vi "Periodic Tasks.vi"(8 "error in (no error)":errorcluster) -> ()   [LabVIEW 2014]
doc: "This VI runs in parallel to other tasks. It can contain as many user-defined periodic loops as you need. These can carry out PID or other sorts of timed response."
uses:
  Variables/References.vi
  <vilib>/Rock Robotics/SystemInterfaces/Utilities/FPGA_UtilitiesRead LocalTime.vi
  Variables/Physical data.vi
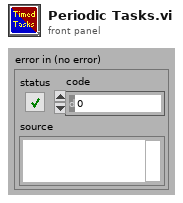
[diagram p1: front panel]
types:
  T1 = typedef "WPI_MotorControlDeviceRef.ctl" = cluster{"DeviceStatus":errorcluster, "Type":T2, "PWM":cluster{"Controller":T3, "PWM Channel":T4, "DeadBand":T5}, "CAN":cluster{"Device Number":u8, "Control Mode":T6, "Semaphore":T7, "Max Vout":dbl, "TalonSRX Control Mode":T8}, "Invert":bool, "TransformRef":T9, "InvTransformRef":T9}
  T2 = typedef "WPI_MotorControlType.ctl" = enum16{"PWM", "CAN", "CANTalonSRX"}
  T3 = typedef "FPGA_TypedefDigitalModule.ctl" = enum16{"Controller 1"}
  T4 = typedef "FPGA_DIOPWMChannel.ctl" = enum8{"PWM 0", "PWM 1", "PWM 2", "PWM 3", "PWM 4", "PWM 5", "PWM 6", "PWM 7", "PWM 8", "PWM 9", "PWM MXP 0", "PWM MXP 1", "PWM MXP 2", "PWM MXP 3", "PWM MXP 4", "PWM MXP 5", "PWM MXP 6", "PWM MXP 7", "PWM MXP 8", "PWM MXP 9", "Invalid"}
  T5 = typedef "WPI_PWMDeadband.ctl" = cluster{"Name":string, "maxPositivePwm":i32, "minPositivePwm":i32, "centerPwm":i32, "maxNegativePwm":i32, "minNegativePwm":i32, "angularRange":u16}
  T6 = typedef "WPI_CANJaguar_ControlMode.ctl" = enum8{"Percent VBus", "Current", "Speed", "Position", "Voltage"}
  T7 = typedef "Semaphore RefNum" = refnum<k1>
  T8 = typedef "WPI_CANTalonSRX_APIControlMode.ctl" = enum8{"Percent VBus", "Speed", "Position", "Slave", "Unchanged / Invalid"}
  T9 = typedef "WPI_PWMTransform_ConPane.ctl" = refnum<vi>
  T10 = typedef "WPI_AnalogChannelDevRef.ctl" = cluster{"DevStatus":errorcluster, "Controller":T11, "Analog Channel":T12}
  T11 = typedef "FPGA_TypedefAnalogModule.ctl" = enum16{"Controller 1"}
  T12 = typedef "FPGA_AIChannel.ctl" = enum8{"AI 0", "AI 1", "AI 2", "AI 3", "AI MXP 0", "AI MXP 1", "AI MXP 2", "AI MXP 3", "Invalid"}
  T13 = typedef "WPI_EncoderDevRef.ctl" = cluster{"DevStatus":errorcluster, "EncoderIndex":T14, "CounterIndex":T15, "DistancePerCount":dbl, "Decoding Type":T16}
  T14 = typedef "FPGA_EncoderIdx.ctl" = enum8{"Enc 0", "Enc 1", "Enc 2", "Enc 3", "Enc 4", "Enc 5", "Enc 6", "Enc 7", "Invalid"}
  T15 = typedef "FPGA_CounterCtrSystemIndex.ctl" = enum8{"Ctr 0", "Ctr 1", "Ctr 2", "Ctr 3", "Ctr 4", "Ctr 5", "Ctr 6", "Ctr 7", "Invalid"}
  T16 = typedef "WPI_EncoderType.ctl" = enum16{"1x", "2x", "4x"}
  T17 = cluster{"DriveMotorRef":T1, "TurretMotorRef":T1, "Turret Encoder":cluster{"AIDeviceRef":T10, "Turret Analog Location":enum16{"RoboRio", "Drive SRX", "Turret SRX"}}, "Drive Encoder":cluster{"EncoderDevRef":T13, "Drive Encoder Location":enum16{"RoboRio", "Drive SRX", "Turret SRX"}}, "Pod position (RCS)":cluster{"X":dbl, "Y":dbl, "Z":dbl}, "Data":cluster{"Drive Motor Output":dbl, "Turret Motor Output":dbl, "Wheel RPM":dbl, "Turret Angle":dbl, "Turret angle offset":dbl, "Transmission moment of inertia":dbl, "Transmission efficiency":dbl, "Wheel dist / rev":dbl, "Turret moment of inertia":dbl, "Inv. turret encoder":bool, "Inv. drive encoder":bool}}[]
  T18 = typedef "NI_Matrix.lvlib/RealMatrix.ctl" = dbl[][]
  T19 = cluster{"All pods":cluster{"Drive":cluster{"Drive Motor Output":dbl, "Wheel RPM":dbl, "Linear speed":dbl, "Linear acceleration":dbl, "Encoder Output":dbl}, "Turret":cluster{"Turret Motor Output":dbl, "Turret Angle":dbl, "Turret velocity":dbl, "Turret acceleration":dbl, "Encoder Output":dbl}, "Pod position (RCS)":cluster{"X":dbl, "Y":dbl, "Z":dbl}}[], "Global Robot Data":cluster{"Position Data":cluster{"Robot Position":cluster{"X":dbl, "Y":dbl, "Z":dbl}, "Robot Velocity":cluster{"X":dbl, "Y":dbl, "Z":dbl}, "Robot Acceleration":cluster{"X":dbl, "Y":dbl, "Z":dbl}}, "Rotation Data":cluster{"Angular Position":cluster{"X":dbl, "Y":dbl, "Z":dbl}, "Angular Velocity":cluster{"X":dbl, "Y":dbl, "Z":dbl}, "Angular Acceleration":cluster{"X":dbl, "Y":dbl, "Z":dbl}}}, "Inertial Characteristics":cluster{"Center of Mass (RCS)":cluster{"X":dbl, "Y":dbl, "Z":dbl}, "Mass Elements":cluster{"X":dbl, "Y":dbl, "Z":dbl, "Mass":dbl, "Name":string}[], "Center of Rotation (RCS)":cluster{"X":dbl, "Y":dbl, "Z":dbl}, "Tensor of Inertia":T18}}
  T20 = cluster{"Drive":cluster{"Drive Motor Output":dbl, "Wheel RPM":dbl, "Linear speed":dbl, "Linear acceleration":dbl, "Encoder Output":dbl}, "Turret":cluster{"Turret Motor Output":dbl, "Turret Angle":dbl, "Turret velocity":dbl, "Turret acceleration":dbl, "Encoder Output":dbl}, "Pod position (RCS)":cluster{"X":dbl, "Y":dbl, "Z":dbl}}
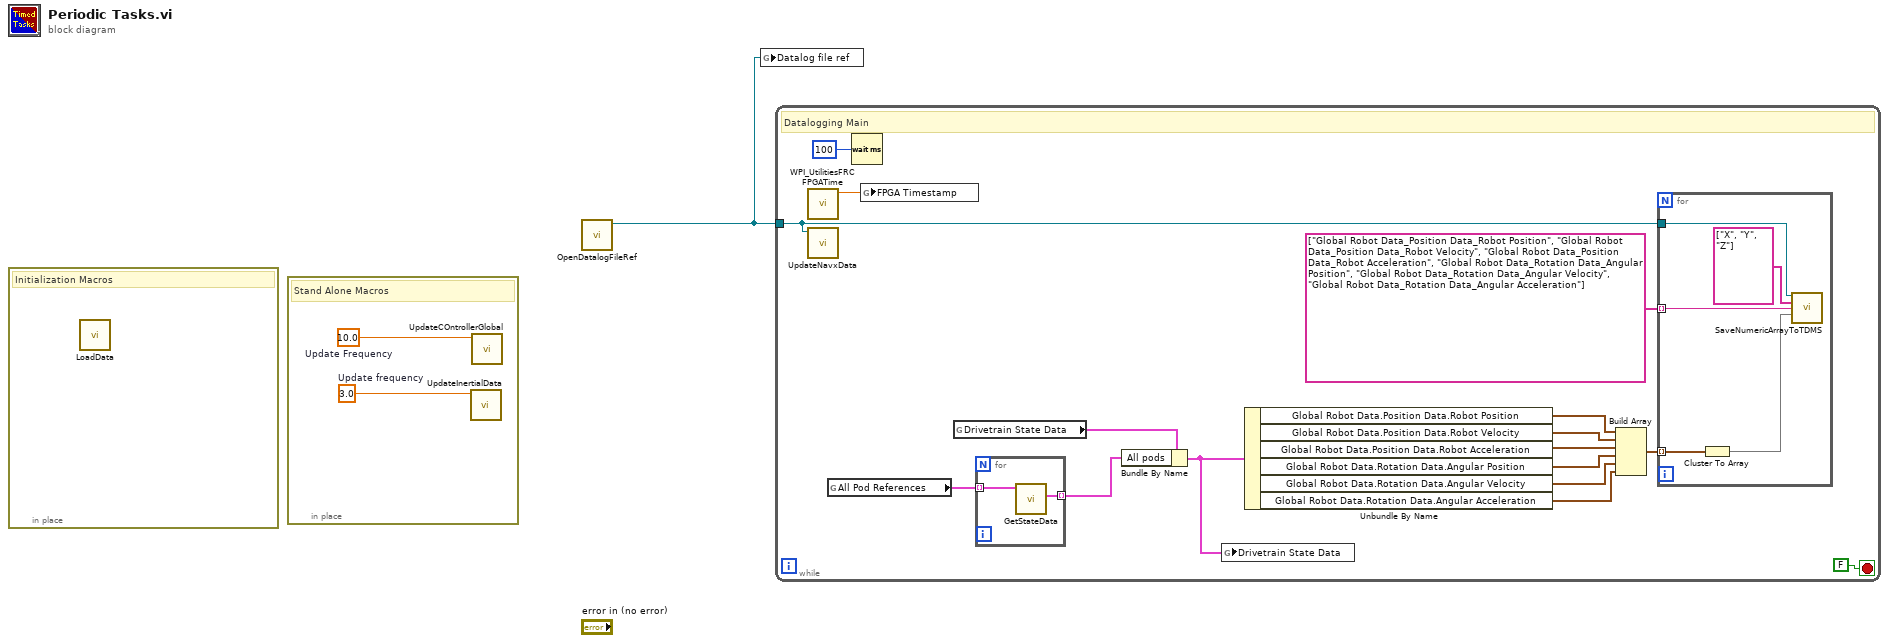
[diagram p0: block diagram]
diagram:
  n1 = in-place {
    # "Initialization Macros"
    n2 = call "LoadData.vi"() -> ()  [unwired: 12 in]
  }
  n3 = in-place {
    w2 = 3.0  # Update frequency
    w3 = 10.0  # Update Frequency
    # "Stand Alone Macros"
    n4 = call "UpdateInertialData.vi"("Update frequency"=w2) -> ()  [unwired: 11 in]
    n5 = call "UpdateCOntrollerGlobal.vi"("Update Frequency"=w3) -> ()  [unwired: 11 in]
  }
  n6 = call "OpenDatalogFileRef.vi"() -> ("tdms file out"=w1:refnum<k34>)  [unwired: 9 in, 2 out]
  n7 = global write "References.vi" "Datalog file ref"(w1) -> ()
  n8 = while {
    tunnel: w1 -> [w4]
    stop <- FALSE stop-if-true
    # "Datalogging Main"
    n9 = call <vilib>:"WPI_UtilitiesFRC FPGATime.vi"() -> ("FPGA Time"=w13:dbl)  [unwired: 10 in, 1 out]
    n10 = call "UpdateNavxData.vi"("Datalogging File Refnum in"=w4) -> ()  [unwired: 11 in]
    n11 = global read "References.vi" "All Pod References"() -> (w18:T17)
    n12 = Wait (ms)(milliseconds to wait=u32 100) -> ()  [unwired: 1 out]
    n13 = global write "Physical data.vi" "FPGA Timestamp"(w13) -> ()
    n14 = global read "Physical data.vi" "Drivetrain State Data"() -> (w14:T19)
    n15 = for {
      tunnel: w18 -> [w26] mode=indexing
      tunnel: [w25] -> w17 mode=indexing
      n16 = call "GetStateData.vi"("Pod in"=w26) -> ("Pod States"=w25:T20)  [unwired: 9 in, 1 out]
    }
    n17 = Bundle By Name(cluster=w14, "All pods"=w17) -> (w15:T19)
    n18 = global write "Physical data.vi" "Drivetrain State Data"(w15) -> ()
    n19 = Unbundle By Name(w15) -> ("Global Robot Data.Position Data.Robot Position"=w12:cluster{"X":dbl, "Y":dbl, "Z":dbl}, "Global Robot Data.Position Data.Robot Velocity"=w11:cluster{"X":dbl, "Y":dbl, "Z":dbl}, "Global Robot Data.Position Data.Robot Acceleration"=w10:cluster{"X":dbl, "Y":dbl, "Z":dbl}, "Global Robot Data.Rotation Data.Angular Position"=w9:cluster{"X":dbl, "Y":dbl, "Z":dbl}, "Global Robot Data.Rotation Data.Angular Velocity"=w8:cluster{"X":dbl, "Y":dbl, "Z":dbl}, "Global Robot Data.Rotation Data.Angular Acceleration"=w7:cluster{"X":dbl, "Y":dbl, "Z":dbl})
    n20 = Build Array(w12, w11, w10, w9, w8, w7) -> (w6:cluster{"X":dbl, "Y":dbl, "Z":dbl}[])
    n21 = for {
      tunnel: w6 -> [w22] mode=indexing
      tunnel: string[] ["Global Robot Data_Position Data_Robot Position", "Global Robot Data_Position Data_Robot Velocity", "Global Robot Data_Position Data_Robot Acceleration", "Global Robot Data_Rotation Data_Angular Position", "Global Robot Data_Rotation Data_Angular Velocity", "Global Robot Data_Rotation Data_Angular Acceleration"] ("Array of Channels") -> [w20] mode=indexing
      tunnel: w4 -> [w23]
      n22 = Cluster To Array(cluster=w22) -> (array=w21:dbl[])
      n23 = call "SaveNumericArrayToTDMS.vi"("tdms file ref in"=w23, "Array of Channels"=string[] ["X", "Y", "Z"], "Group Name"=w20, "Array of Values"=w21) -> ()  [unwired: 10 in, 2 out]
    }
  }
